vi "Example.vi"() -> ()   [LabVIEW 2025]
uses:
  <vilib>/numeric/Random Number (Range) I64.vi
  <vilib>/numeric/sub_Random U32.vi
  FastTreeView/Write Column Headers.vi
  FastTreeView/LogDebug--callback.vi
  FastTreeView/FastTreeView.lvclass
  C:/Git/FastTreeView/FastTreeView/LV/FastTreeView/dll/FastTreeView.dll
  FastTreeView/dll/FastTreeView.dll
panel:
  out "element":string
  in  "Collapse All":bool
  in  "Expand All":bool
  out "error out 2":errorcluster
  out "IsGlyph":bool
  out "IsExpander":bool
  out "Tag":string
  out "Column":i32
  in  "Focus on New":bool
  in  "stop":bool
  out "error out":errorcluster
  in  "LvTreeGrid":refnum<k24>(container)
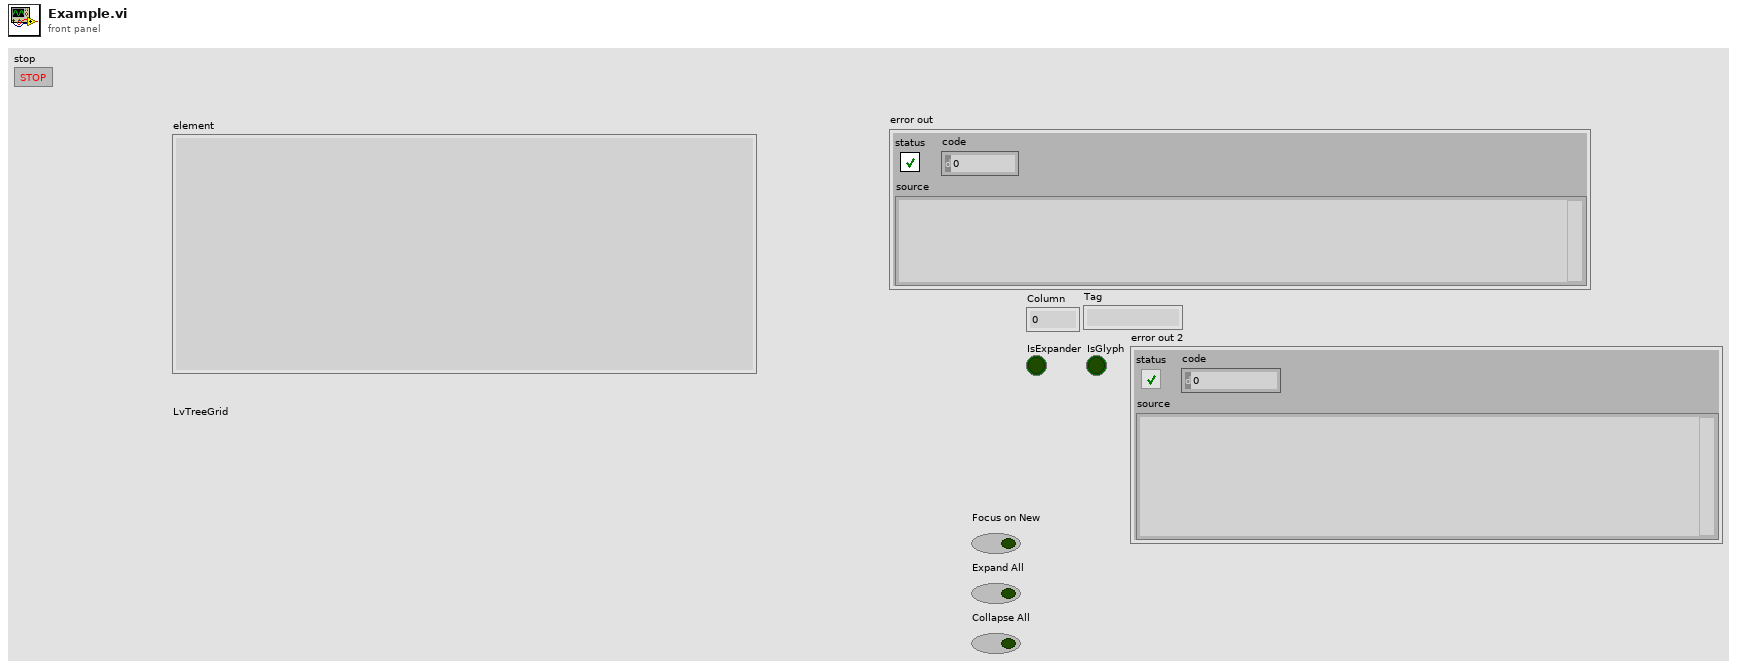
[diagram p1: front panel]
types:
  T1 = cluster{"Left Cell String":string, "Child Text":string[], "Child Tag":string, "Item Indent":i32, "Child Only?":bool, "Glyph Index":i32}
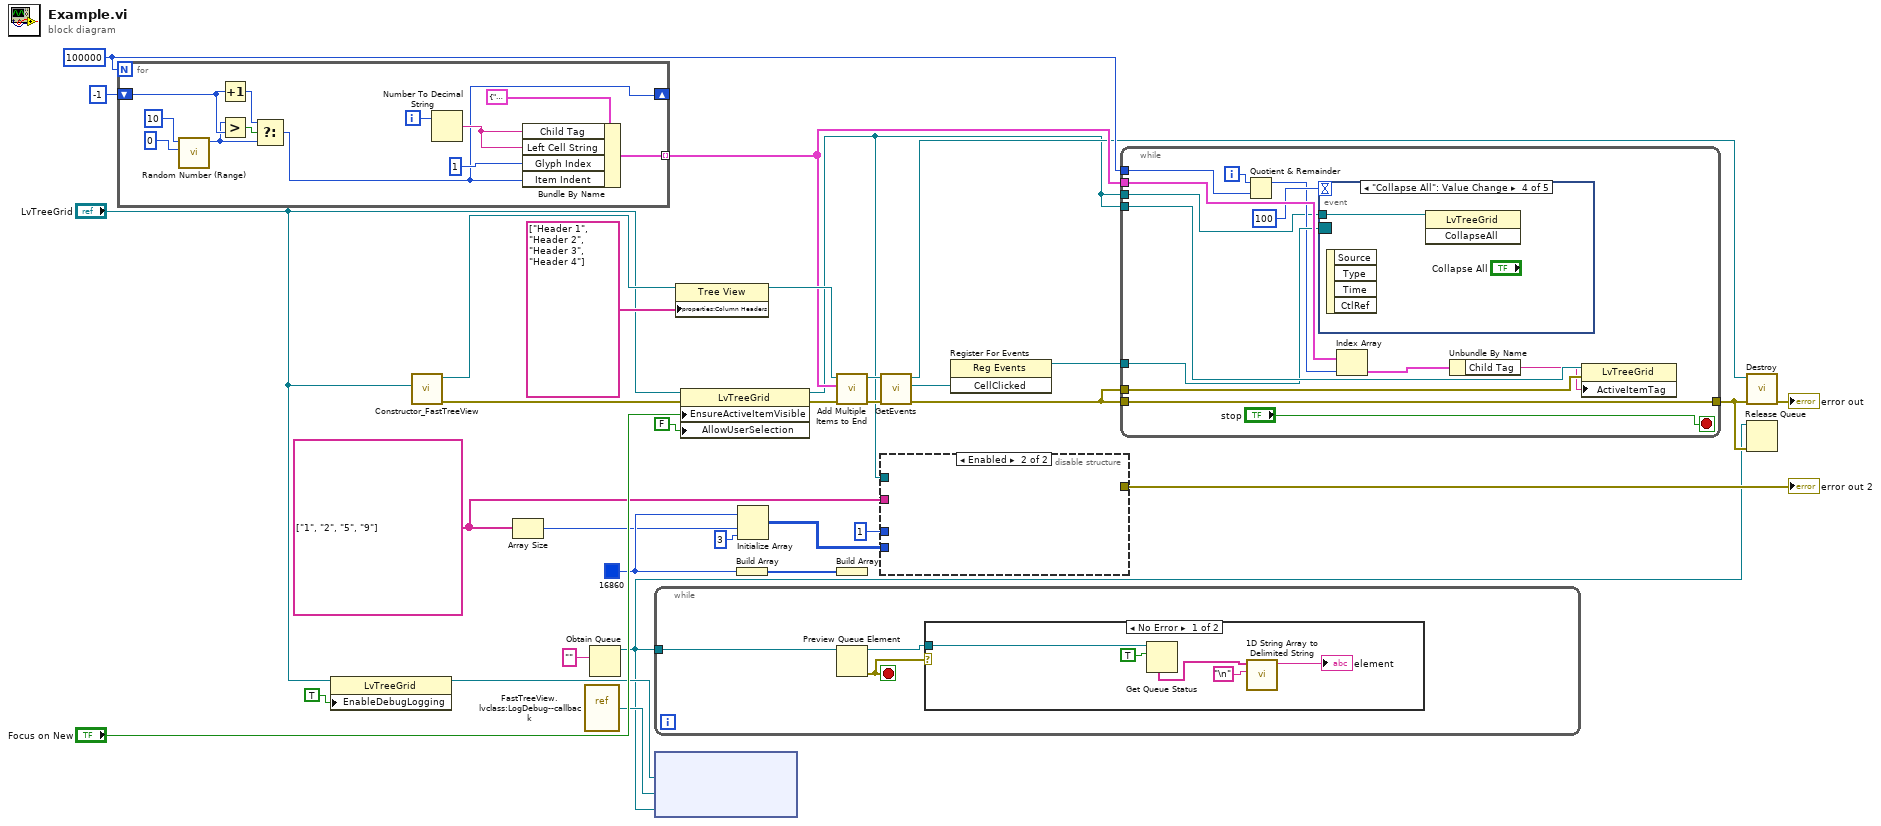
[diagram p0: block diagram]
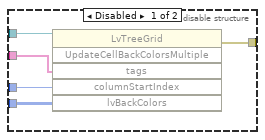
[diagram p3: hidden frame]
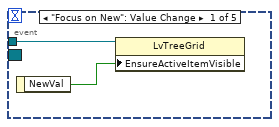
[diagram p4: hidden frame]
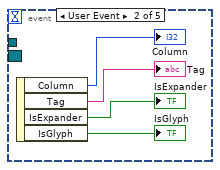
[diagram p5: hidden frame]
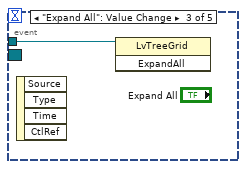
[diagram p6: hidden frame]
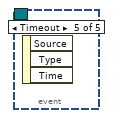
[diagram p7: hidden frame]
diagram:
  w16 = u32 16860
  w17 = string[] ["1", "2", "5", "9"] ("tags")
  w27 = 100000
  n1 = for {
    N: w27 -> [_]
    tunnel: [w44] -> w25 mode=indexing
    shift-right: [w34] -> _
    shift-left: i64 -1 -> [w38]
    i -> [w41]
    n2 = call-poly <vilib>:"Random Number (Range).vi"("lower bound (-100)"=i64 0, "upper bound (100)"=i64 10) -> ("number"=w36:i64)  [unwired: 9 in]
    n3 = Increment(x=w38) -> (x+1=w37:i64)
    n4 = Greater?(x=w36, y=w38) -> (0:w39:bool)
    n5 = Select(t=w37, s=w39, f=w36) -> (s? t:f=w34:i64)
    n6 = Number To Decimal String(number=w41) -> (decimal integer string=w42:string)  [unwired: 1 in]
    n7 = Bundle By Name(cluster=T1 {"Left Cell String"="", "Child Text"=[], "Child Tag"="", "Item Indent"=0, "Child Only?"=FALSE, "Glyph Index"=0} ("Item"), "Child Tag"=w42, "Left Cell String"=w42, "Glyph Index"=1, "Item Indent"=w34) -> (w44:T1)
  }
  n8 = property class="LvTreeGrid"(reference="LvTreeGrid", "EnableDebugLogging"=TRUE) -> (reference out=w6:refnum<k24>)  [unwired: 1 in, 1 out]
  n9 = call "Constructor_FastTreeView.vi"("LvTreeGrid"="LvTreeGrid") -> ("error out"=w10:errorcluster, "FastTreeView out"=w31:refnum<class "FastTreeView.lvclass">)  [unwired: 9 in]
  n10 = Array Size(array=w17) -> (size(s)=w13:i32)
  n11 = vi-ref "FastTreeView.lvclass:LogDebug--callback.vi"() -> ("vi reference"=w3:refnum<vi>)
  n12 = Obtain Queue(element data type="") -> (queue out=w1:refnum<queue>)  [unwired: 4 in, 2 out]
  n13 = while {
    tunnel: w1 -> [w48]
    stop <- w46 stop-if-true
    n14 = Preview Queue Element(queue=w48) -> (queue out=w47:refnum<queue>, error out=w46:errorcluster)  [unwired: 2 in, 2 out]
    n15 = case shown="No Error" w46 {
      tunnel: w47 -> [w53 _]
      frame No Error {
        n16 = Get Queue Status(queue=w53, return elements? (F)=TRUE) -> (elements=w51:string[])  [unwired: 1 in, 7 out]
        n17 = call <vilib>:"1D String Array to Delimited String.vi"("delimiter"="\n", "string array"=w51) -> ("delimited string"=→"element":string)  [unwired: 9 in]
      }
      frame Error {
      }
    }
  }
  n18 = node(w6, w3, w1) -> ()  [unwired: 2 in, 2 out]
  n19 = property class="Tree View"(reference=w31, "properties:Column Headers"=string[] ["Header 1", "Header 2", "Header 3", "Header 4"] ("Column Headers")) -> (reference out=w32:refnum<class "FastTreeView.lvclass">)  [unwired: 1 in, 1 out]
  n20 = property class="LvTreeGrid"(reference="LvTreeGrid", error in=w10, "EnsureActiveItemVisible"="Focus on New", "AllowUserSelection"=FALSE ("Enabled")) -> (reference out=w11:refnum<k24>, error out=w9:errorcluster)
  n21 = Build Array(w16) -> (w29:u32[])
  n22 = Initialize Array(w16, w13, 3 ("dimension size")) -> (w15:u32[][])
  n23 = call "Add Multiple Items to End.vi"("error in (no error)"=w9, "Items"=w25, "FastTreeView in"=w32) -> ("error out"=w18:errorcluster, "FastTreeView out"=w21:refnum<class "FastTreeView.lvclass">)  [unwired: 7 in]
  n24 = Build Array(w29) -> ()  [unwired: 1 out]
  n25 = call "GetEvents.vi"("error in (no error)"=w18, "Tree View in"=w21) -> ("error out"=w8:errorcluster, "CellClicked"=w19:refnum<user-event>, "Tree View out"=w20:refnum<class "FastTreeView.lvclass">)  [unwired: 7 in]
  n26 = disable-structure shown="Enabled" {
    disable-tunnel: 1 ("columnStartIndex") -> [w58 _]
    disable-tunnel: w11 -> [w57 _]
    disable-tunnel: w17 -> [w56 _]
    disable-tunnel: w15 -> [w55 _]
    disable-tunnel: [w54 _] -> w14
    frame Disabled {
      n27 = invoke class="LvTreeGrid" method="UpdateCellBackColorsMultiple"(reference=w57, "tags"=w56, "columnStartIndex"=w58, "lvBackColors"=w55) -> (error out=w54:errorcluster)  [unwired: 2 in, 5 out]
    }
    frame Enabled {
    }
  }
  "error out 2" <- w14
  n28 = register-events(w19) -> (reference out=w24:refnum<event-registration>)  [unwired: 2 in, 1 out]
  n29 = while {
    tunnel: w8 -> [w71]
    tunnel: [w71] -> w2
    tunnel: w11 -> [w70]
    tunnel: w8 -> [w69]
    tunnel: w25 -> [w68]
    tunnel: w27 -> [w66]
    tunnel: w24 -> [w64]
    tunnel: w11 -> [w59]
    i -> [w67]
    stop <- "stop" stop-if-true
    n30 = Quotient & Remainder(x=w67, y=w66) -> (x-y*floor(x/y)=w61:i32)  [unwired: 1 out]
    n31 = event shown="[3] \"Collapse All\": Value Change" {
      selector: w64 -> [_ _ _ _ _]
      dyn-events: _ -> [_ _ _ _ _]
      timeout: 100 -> [_ _ _ _ _]
      tunnel: w59 -> [w73 _ w78 w79 _]
      event "Focus on New": Value Change {
        n32 = event-data() -> ("NewVal"=w72:bool)  [unwired: 1 in]
        n33 = property class="LvTreeGrid"(reference=w73, "EnsureActiveItemVisible"=w72) -> ()  [unwired: 1 in, 2 out]
      }
      event User Event {
        n34 = event-data() -> ("Column"=→"Column":i32, "Tag"=→"Tag":string, "IsExpander"=→"IsExpander":bool, "IsGlyph"=→"IsGlyph":bool)  [unwired: 1 in]
      }
      event "Expand All": Value Change {
        n35 = event-data() -> ()  [unwired: 1 in, 4 out]
        n36 = invoke class="LvTreeGrid" method="ExpandAll"(reference=w78) -> ()  [unwired: 2 in, 3 out]
      }
      event "Collapse All": Value Change {
        n37 = event-data() -> ()  [unwired: 1 in, 4 out]
        n38 = invoke class="LvTreeGrid" method="CollapseAll"(reference=w79) -> ()  [unwired: 2 in, 3 out]
      }
      event Timeout {
        n39 = event-data() -> ()  [unwired: 1 in, 3 out]
      }
    }
    n40 = Index Array(array=w68, index=w61) -> (element=w62:T1)
    n41 = Unbundle By Name(w62) -> ("Child Tag"=w60:string)
    n42 = property class="LvTreeGrid"(reference=w70, error in=w69, "ActiveItemTag"=w60) -> ()  [unwired: 2 out]
  }
  n43 = call "Destroy.vi"("error in (no error)"=w2, "FastTreeView in"=w20) -> ("error out"=→"error out":errorcluster)  [unwired: 8 in, 1 out]
  n44 = Release Queue(queue=w1, error in (no error)=w2) -> ()  [unwired: 1 in, 3 out]
